vi "Atenuate Color.vi"(10 "Gain":sgl, 11 "Color In":u32(colorbox)) -> (3 "Color Out":u32(colorbox))   [LabVIEW 2019, in "Display Utilities.lvlib"]
uses:
  Display Utilities.lvlib
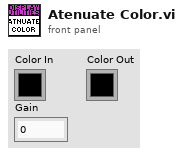
[diagram p1: front panel]
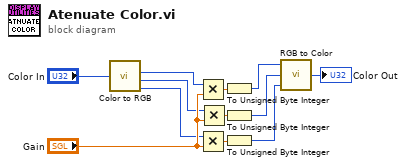
[diagram p0: block diagram]
diagram:
  n1 = call <vilib>:"Color to RGB.vi"("Color"="Color In") -> ("R"=w10:u8, "G"=w9:u8, "B"=w8:u8)  [unwired: 1 out]
  n2 = Multiply(x=w10, y="Gain") -> (x*y=w4:sgl)
  n3 = Multiply(x=w8, y="Gain") -> (x*y=w5:sgl)
  n4 = Multiply(x=w9, y="Gain") -> (x*y=w6:sgl)
  n5 = To Unsigned Byte Integer(number=w4) -> (unsigned 8bit integer=w3:u8)
  n6 = To Unsigned Byte Integer(number=w6) -> (unsigned 8bit integer=w2:u8)
  n7 = To Unsigned Byte Integer(number=w5) -> (unsigned 8bit integer=w1:u8)
  n8 = call <vilib>:"RGB to Color.vi"("B"=w1, "G"=w2, "R"=w3) -> ("Color"=→"Color Out":u32)
